vi "Thermometer (Demo).vi"(8 "에러 입력(에러 없음)":errorcluster, 10 "온도 스케일":bool) -> (0 "에러 출력":errorcluster, 2 "온도":dbl(slide) scale=0.0..100.0 scale format="%.1f")   [LabVIEW 2010]
doc: "이 VI는 DAQ 신호 장치에서 온도 센서를 사용하여 온도를 측정하는 것을 시뮬레이션합니다.\n\nDAQ 보드나 DAQ 신호 장치를 가지고 있다면, 대신에 Thermometer VI를 사용합니다."
panel:
  # "섭씨\n\n화씨"
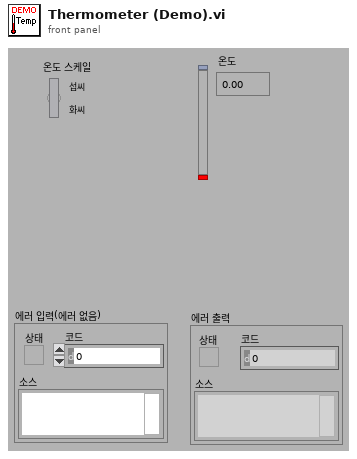
[diagram p1: front panel]
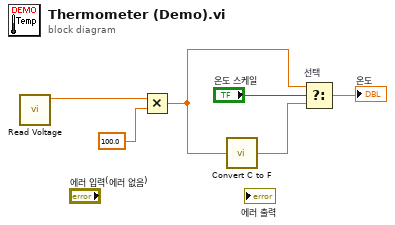
[diagram p0: block diagram]
diagram:
  n1 = call "Read Voltage.vi"() -> ("전압"=w1:dbl)  [unwired: 6 in, 1 out]
  n2 = Multiply(x=w1, y=100.0) -> (x*y=w2:dbl)
  n3 = call "Convert C to F.vi"("섭씨"=w2) -> ("화씨"=w5:dbl)
  n4 = Select "선택"(t=w2, s="온도 스케일", f=w5) -> (s? t:f=→"온도":dbl)
